vi "Questionable Data Status.vi"(6 "Questionable Register Value To Set (0)":i32, 7 "Questionable Register To Set(0: Calibration Status Enable)":i32(ring) items=["Calibration Status Enable", "Calibration Status NTR", "Calibration Status PTR", "Current Status Enable", "Current Status NTR", "Current Status PTR", "Temperature Status Enable", "Temperature Status NTR", "Temperature Status PTR", "Test Status Enable", "Test Status NTR", "Test Status PTR", "Voltage Status Enable", "Voltage Status NTR", "Voltage Status PTR", "Overall Status Enable", "Overall Status NTR", "Overall Status PTR"], 8 "error in (no error)":errorcluster, 9 "Questionable Register To Check (0: Calibration Status Condition)":i32(ring) items=["Calibration Status Condition", "Calibration Status Enable", "Calibration Status Event", "Calibration Status NTR", "Calibration Status PTR", "Current Status Condition", "Current Status Enable", "Current Status Event", "Current Status NTR", "Current Status PTR", "Temperature Status Condition", "Temperature Status Enable", "Temperature Status Event", "Temperature Status NTR", "Temperature Status PTR", "Test Status Condition", "Test Status Enable", "Test Status Event", "Test Status NTR", "Test Status PTR", "Voltage Status Condition", "Voltage Status Enable", "Voltage Status Event", "Voltage Status NTR", "Voltage Status PTR", "Overall Status Condition", "Overall Status Enable", "Overall Status Event", "Overall Status NTR", "Overall Status PTR"], 10 "Operation Mode (0: Check)":i32(ring) items=["Check", "Set"], 11 "VISA resource name":refnum<visa-resource-name>) -> (0 "error out":errorcluster, 2 "Questionable Register Status":bool[](array[boolean]), 3 "VISA resource name out":refnum<visa-resource-name>)   [LabVIEW 2020, in "Agilent B2900 Series.lvlib"]
doc: "Sets or checks the Questionable Data Status registers.\n\n<B>Note:</B> Use this VI only with other low-level VIs. The high-level VIs automatically incorporate this functionality. This VI does not check the instrument status."
uses:
  Agilent B2900 Series.lvlib
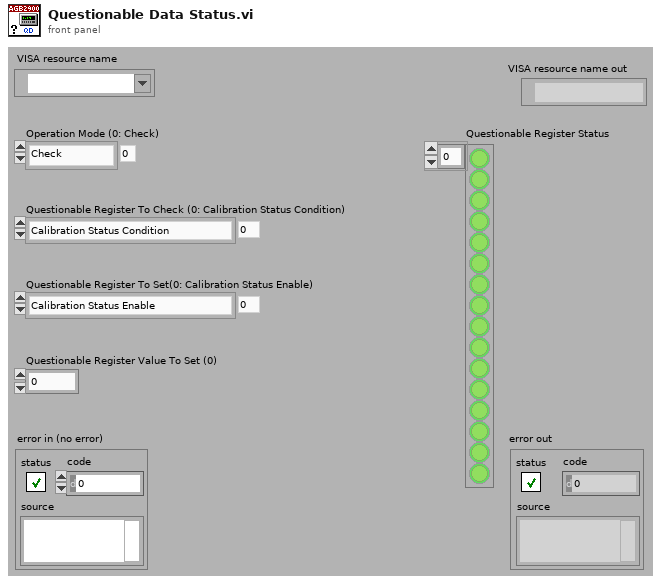
[diagram p1: front panel]
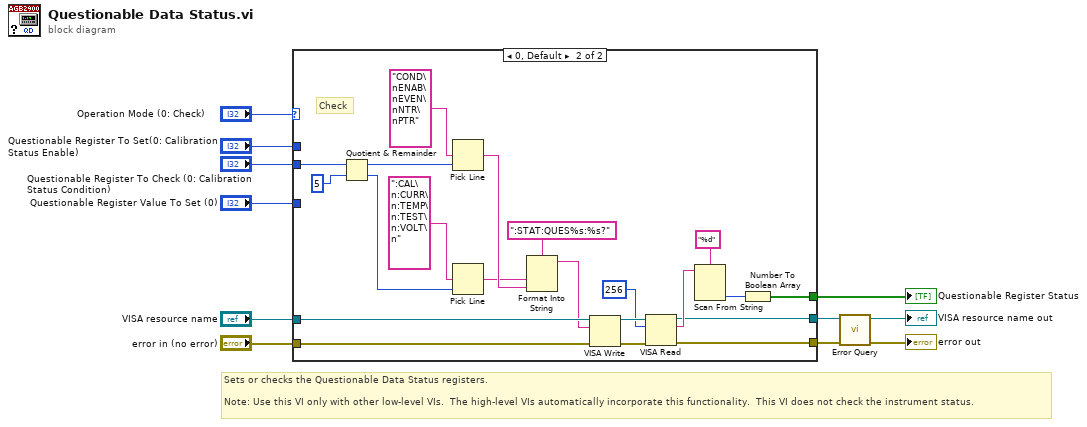
[diagram p0: block diagram]
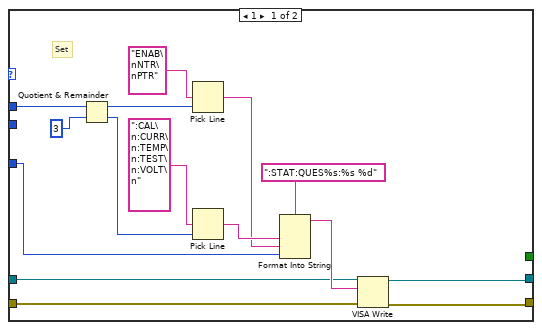
[diagram p2: hidden frame]
diagram:
  # "Sets or checks the Questionable Data Status registers.\n\nNote: Use this VI only with other low-level VIs.  The high-level VIs automatically incorporate this functionality.  This VI does not check the instrument status."
  n1 = case shown="0, Default" "Operation Mode (0: Check)" {
    tunnel: "Questionable Register To Check (0: Calibration Status Condition)" -> [_ w43]
    tunnel: "Questionable Register Value To Set (0)" -> [w18 _]
    tunnel: "VISA resource name" -> [w16 w38]
    tunnel: "error in (no error)" -> [w15 w37]
    tunnel: [_ w30] -> w6
    tunnel: [w14 w29] -> w3
    tunnel: [w13 w28] -> w4
    tunnel: "Questionable Register To Set(0: Calibration Status Enable)" -> [w12 _]
    frame 1 {
      # "Set"
      n2 = Quotient & Remainder(x=w12, y=3) -> (x-y*floor(x/y)=w25:i32, floor(x/y)=w24:i32)
      n3 = Pick Line(multi-line string="ENAB\nNTR\nPTR", line index=w25) -> (output string=w21:string)  [unwired: 1 in]
      n4 = Pick Line(multi-line string=":CAL\n:CURR\n:TEMP\n:TEST\n:VOLT\n", line index=w24) -> (output string=w26:string)  [unwired: 1 in]
      n5 = Format Into String(format string=":STAT:QUES%s:%s %d", w26, w21, w18) -> (resulting string=w17:string)  [unwired: 2 in, 1 out]
      n6 = VISA Write(VISA resource name=w16, write buffer=w17, error in (no error)=w15) -> (VISA resource name out=w14:refnum<visa-resource-name>, error out=w13:errorcluster)  [unwired: 1 out]
    }
    frame 0, Default {
      # "Check"
      n7 = Quotient & Remainder(x=w43, y=5) -> (x-y*floor(x/y)=w40:i32, floor(x/y)=w41:i32)
      n8 = Pick Line(multi-line string="COND\nENAB\nEVEN\nNTR\nPTR", line index=w40) -> (output string=w45:string)  [unwired: 1 in]
      n9 = Pick Line(multi-line string=":CAL\n:CURR\n:TEMP\n:TEST\n:VOLT\n", line index=w41) -> (output string=w39:string)  [unwired: 1 in]
      n10 = Format Into String(format string=":STAT:QUES%s:%s?", w39, w45) -> (resulting string=w36:string)  [unwired: 2 in, 1 out]
      n11 = VISA Write(VISA resource name=w38, write buffer=w36, error in (no error)=w37) -> (VISA resource name out=w34:refnum<visa-resource-name>, error out=w35:errorcluster)  [unwired: 1 out]
      n12 = VISA Read(VISA resource name=w34, byte count=u32 256, error in (no error)=w35) -> (VISA resource name out=w29:refnum<visa-resource-name>, read buffer=w33:string, error out=w28:errorcluster)  [unwired: 1 out]
      n13 = Scan From String(format string="%d", input string=w33) -> (output 1=w32:i32)  [unwired: 3 in, 3 out]
      n14 = Number To Boolean Array(number=w32) -> (Boolean array=w30:bool[])
    }
  }
  "Questionable Register Status" <- w6
  n15 = call "Error Query.vi"("error in (no error)"=w4, "VISA resource name"=w3) -> ("error out"=→"error out":errorcluster, "VISA resource name out"=→"VISA resource name out":refnum<visa-resource-name>)  [unwired: 6 in, 2 out]
